vi "Dynamic vi.vi"(8 "error in (no error)":errorcluster, 11 "Test Case Test Double in":refnum<class "Test Case Test Double.lvclass">) -> (0 "error out":errorcluster, 3 "Test Case Test Double out":refnum<class "Test Case Test Double.lvclass">)   [LabVIEW 2020, in "Test Case Test Double.lvclass"]
uses:
  Test Case Test Double.lvclass
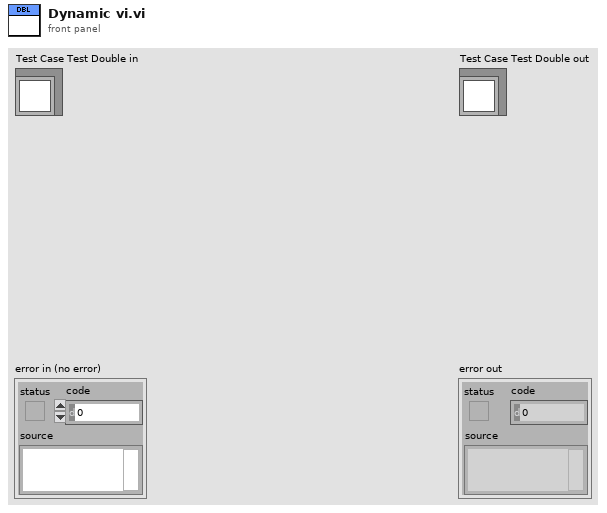
[diagram p1: front panel]
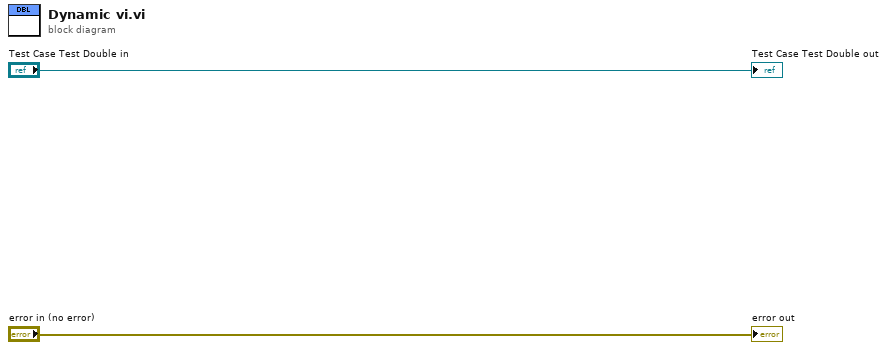
[diagram p0: block diagram]
diagram:
  "error out" <- "error in (no error)"
  "Test Case Test Double out" <- "Test Case Test Double in"
